vi "pidLateral.vi"(7 "PID gains Lateral":cluster{"(Kc)":dbl, "(Ki)":dbl, "(Kd)":dbl}={"(Kc)"=2.0, "(Ki)"=0.0, "(Kd)"=0.3}, 8 "error in (no error)":errorcluster, 11 "Robot in":refnum<class "Robot.lvclass">) -> (0 "error out":errorcluster, 3 "Robot out":refnum<class "Robot.lvclass">)   [LabVIEW 2023, in "Robot.lvclass"]
uses:
  Robot.lvclass
  C:/Users/ebert/Desktop/roboime/SSL_AI/Object_class/Object.lvclass
  Game_class/Navigation/driveMode.ctl
  Robot.lvclass/Robot.ctl
  Object_class/Object.lvclass/Object.ctl
  <vilib>/Analysis/coordinate.llb/2D Cartesian Coordinate Rotation (Scalar).vi
  Read path_smooth.vi
  Object_class/Read x.vi
  Object_class/Read y.vi
  Read orientation.vi
  Read v_tang.vi
  Read v_norm.vi
  Write v_tang.vi
  Write v_norm.vi
  <vilib>/Analysis/NI_AALPro.lvlib
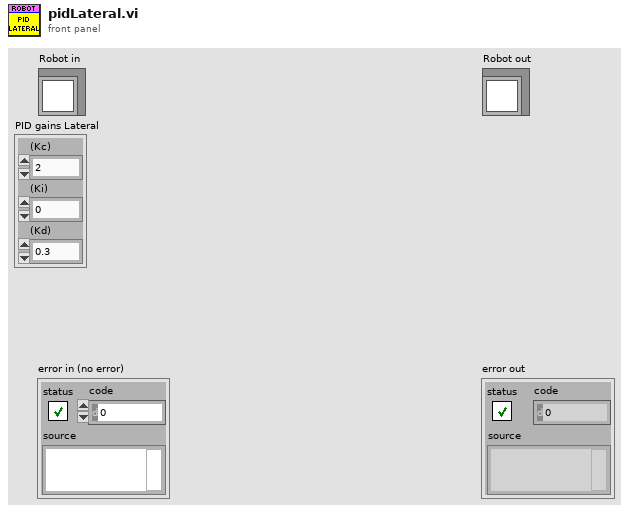
[diagram p1: front panel]
types:
  T1 = typedef "driveMode.ctl" = enum16{"Fast", "SafeDrive"}
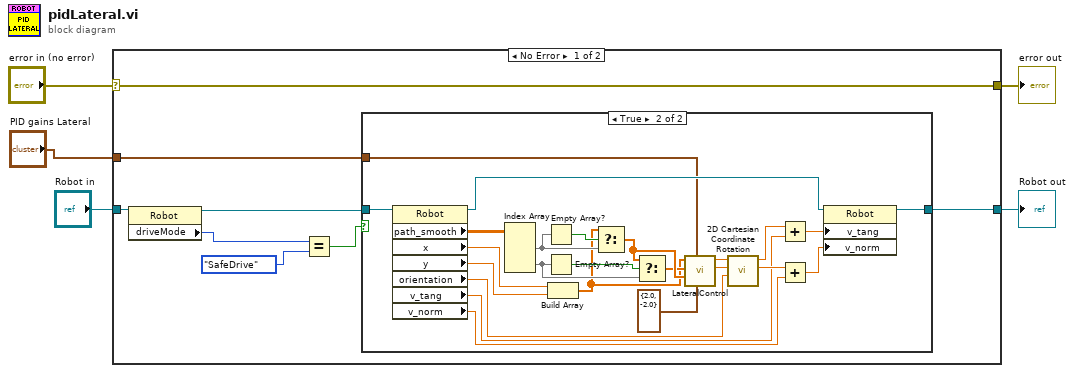
[diagram p0: block diagram]
diagram:
  n1 = case shown="No Error" "error in (no error)" {
    selector: "error in (no error)" -> [w13 w40]
    tunnel: [w13 w40] -> w4
    tunnel: [w12 w39] -> w2
    tunnel: "Robot in" -> [w10 w39]
    tunnel: "PID gains Lateral" -> [w11 _]
    frame No Error {
      n2 = property class="Robot"(reference=w10) -> (reference out=w9:refnum<class "Robot.lvclass">, "driveMode"=w8:T1)  [unwired: 1 in, 1 out]
      n3 = Equal?(x=w8, y=driveMode."SafeDrive") -> (x = y?=w6:bool)
      n4 = case shown="True" w6 {
        tunnel: [w14 w17] -> w12
        tunnel: w11 -> [_ w16]
        tunnel: w9 -> [w14 w15]
        frame False {
        }
        frame True {
          n5 = property class="Robot"(reference=w15) -> (reference out=w28:refnum<class "Robot.lvclass">, "path_smooth"=w34:dbl[][], "x"=w33:dbl, "y"=w32:dbl, "orientation"=w25:dbl, "v_tang"=w22:dbl, "v_norm"=w21:dbl)  [unwired: 1 in, 1 out]
          n6 = Index Array(array=w34) -> (element #1=w35:dbl[], element #2=w37:dbl[])  [unwired: 4 in]
          n7 = Empty Array?(array=w35) -> (empty?=w36:bool)
          n8 = Empty Array?(array=w37) -> (empty?=w38:bool)
          n9 = Build Array(w33, w32) -> (w29:dbl[])
          n10 = Select(t=w29, s=w36, f=w35) -> (s? t:f=w31:dbl[])
          n11 = Select(t=w31, s=w38, f=w37) -> (s? t:f=w30:dbl[])
          n12 = call "LateralControl.vi"("output range"=cluster{"output high":dbl, "output low":dbl} {"output high"=2.0, "output low"=-2.0}, "PID Gains lateral"=w16, "Waypoint 0"=w31, "Waypoint 1"=w30, "Position"=w29) -> ("y out"=w26:dbl, "x out"=w27:dbl)  [unwired: 5 in]
          n13 = call-poly <vilib>:"2D Cartesian Coordinate Rotation.vi"("theta"=w25, "y"=w26, "x"=w27) -> ("y out"=w23:dbl, "x out"=w24:dbl)  [unwired: 6 in, 1 out]
          n14 = Add(x=w24, y=w22) -> (x+y=w20:dbl)
          n15 = Add(x=w23, y=w21) -> (x+y=w19:dbl)
          n16 = property class="Robot"(reference=w28, "v_tang"=w20, "v_norm"=w19) -> (reference out=w17:refnum<class "Robot.lvclass">)  [unwired: 1 in, 1 out]
        }
      }
    }
    frame Error {
    }
  }
  "error out" <- w4
  "Robot out" <- w2
